vi "Set Controls State.vi"(10 "Disabled":T1(ring), 11 "Ctrl Refs":refnum<vi>[](array[refnum])) -> ()   [LabVIEW 2020]
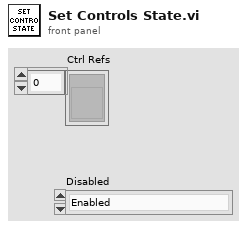
[diagram p1: front panel]
types:
  T1 = enum8{"Enabled", "Disabled", "Disabled and Grayed Out"}
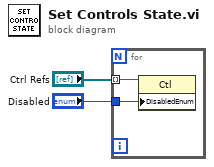
[diagram p0: block diagram]
diagram:
  n1 = for {
    tunnel: "Ctrl Refs" -> [w4] mode=indexing
    tunnel: "Disabled" -> [w3]
    n2 = property class="Ctl"(reference=w4, "DisabledEnum"=w3) -> ()  [unwired: 1 in, 2 out]
  }
